vi "OceanOptics_30sec_img_while_scan.vi"() -> ()   [LabVIEW 2016]
uses:
  C:/Program Files/Ocean Optics/OmniDriver/OOI_HOME/NETOmniDriver-NET40.dll
  Program Files/Ocean Optics/OmniDriver/OOI_HOME/NETOmniDriver-NET40.dll
  <vilib>/DAQmx/create/channels.llb/DAQmx Create Channel (DO-Digital Output).vi
panel:
  in  "lastTriggerMilliseconds":i32
  in  "error in":errorcluster
  out "error out 2":errorcluster
  in  "Trigger":bool
  in  "Action B":bool
  out "getBufferCapacity":i32
  in  "read":bool
  in  "start":bool
  in  "abort":bool
  in  "stop":bool
  out "spectrum":cluster{"Y":dbl[], "Y":dbl[]}[](graph)
  out "getExternalTriggerMode":i32
  in  "clear":bool
  out "getNumberOfElements before readout":i32
  out "status":bool
  out "error out":errorcluster
  in  "integration time [us]":i32=100000
  # "Mode 3 = single trigger"
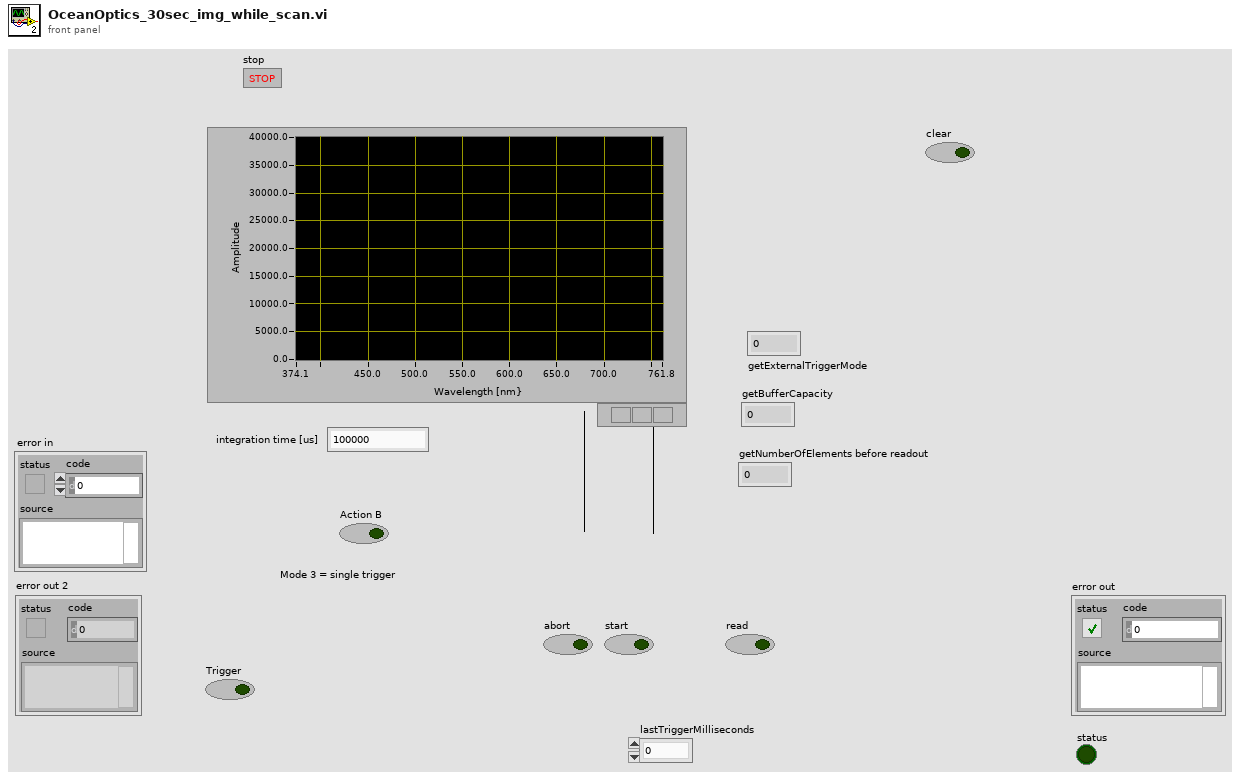
[diagram p1: front panel]
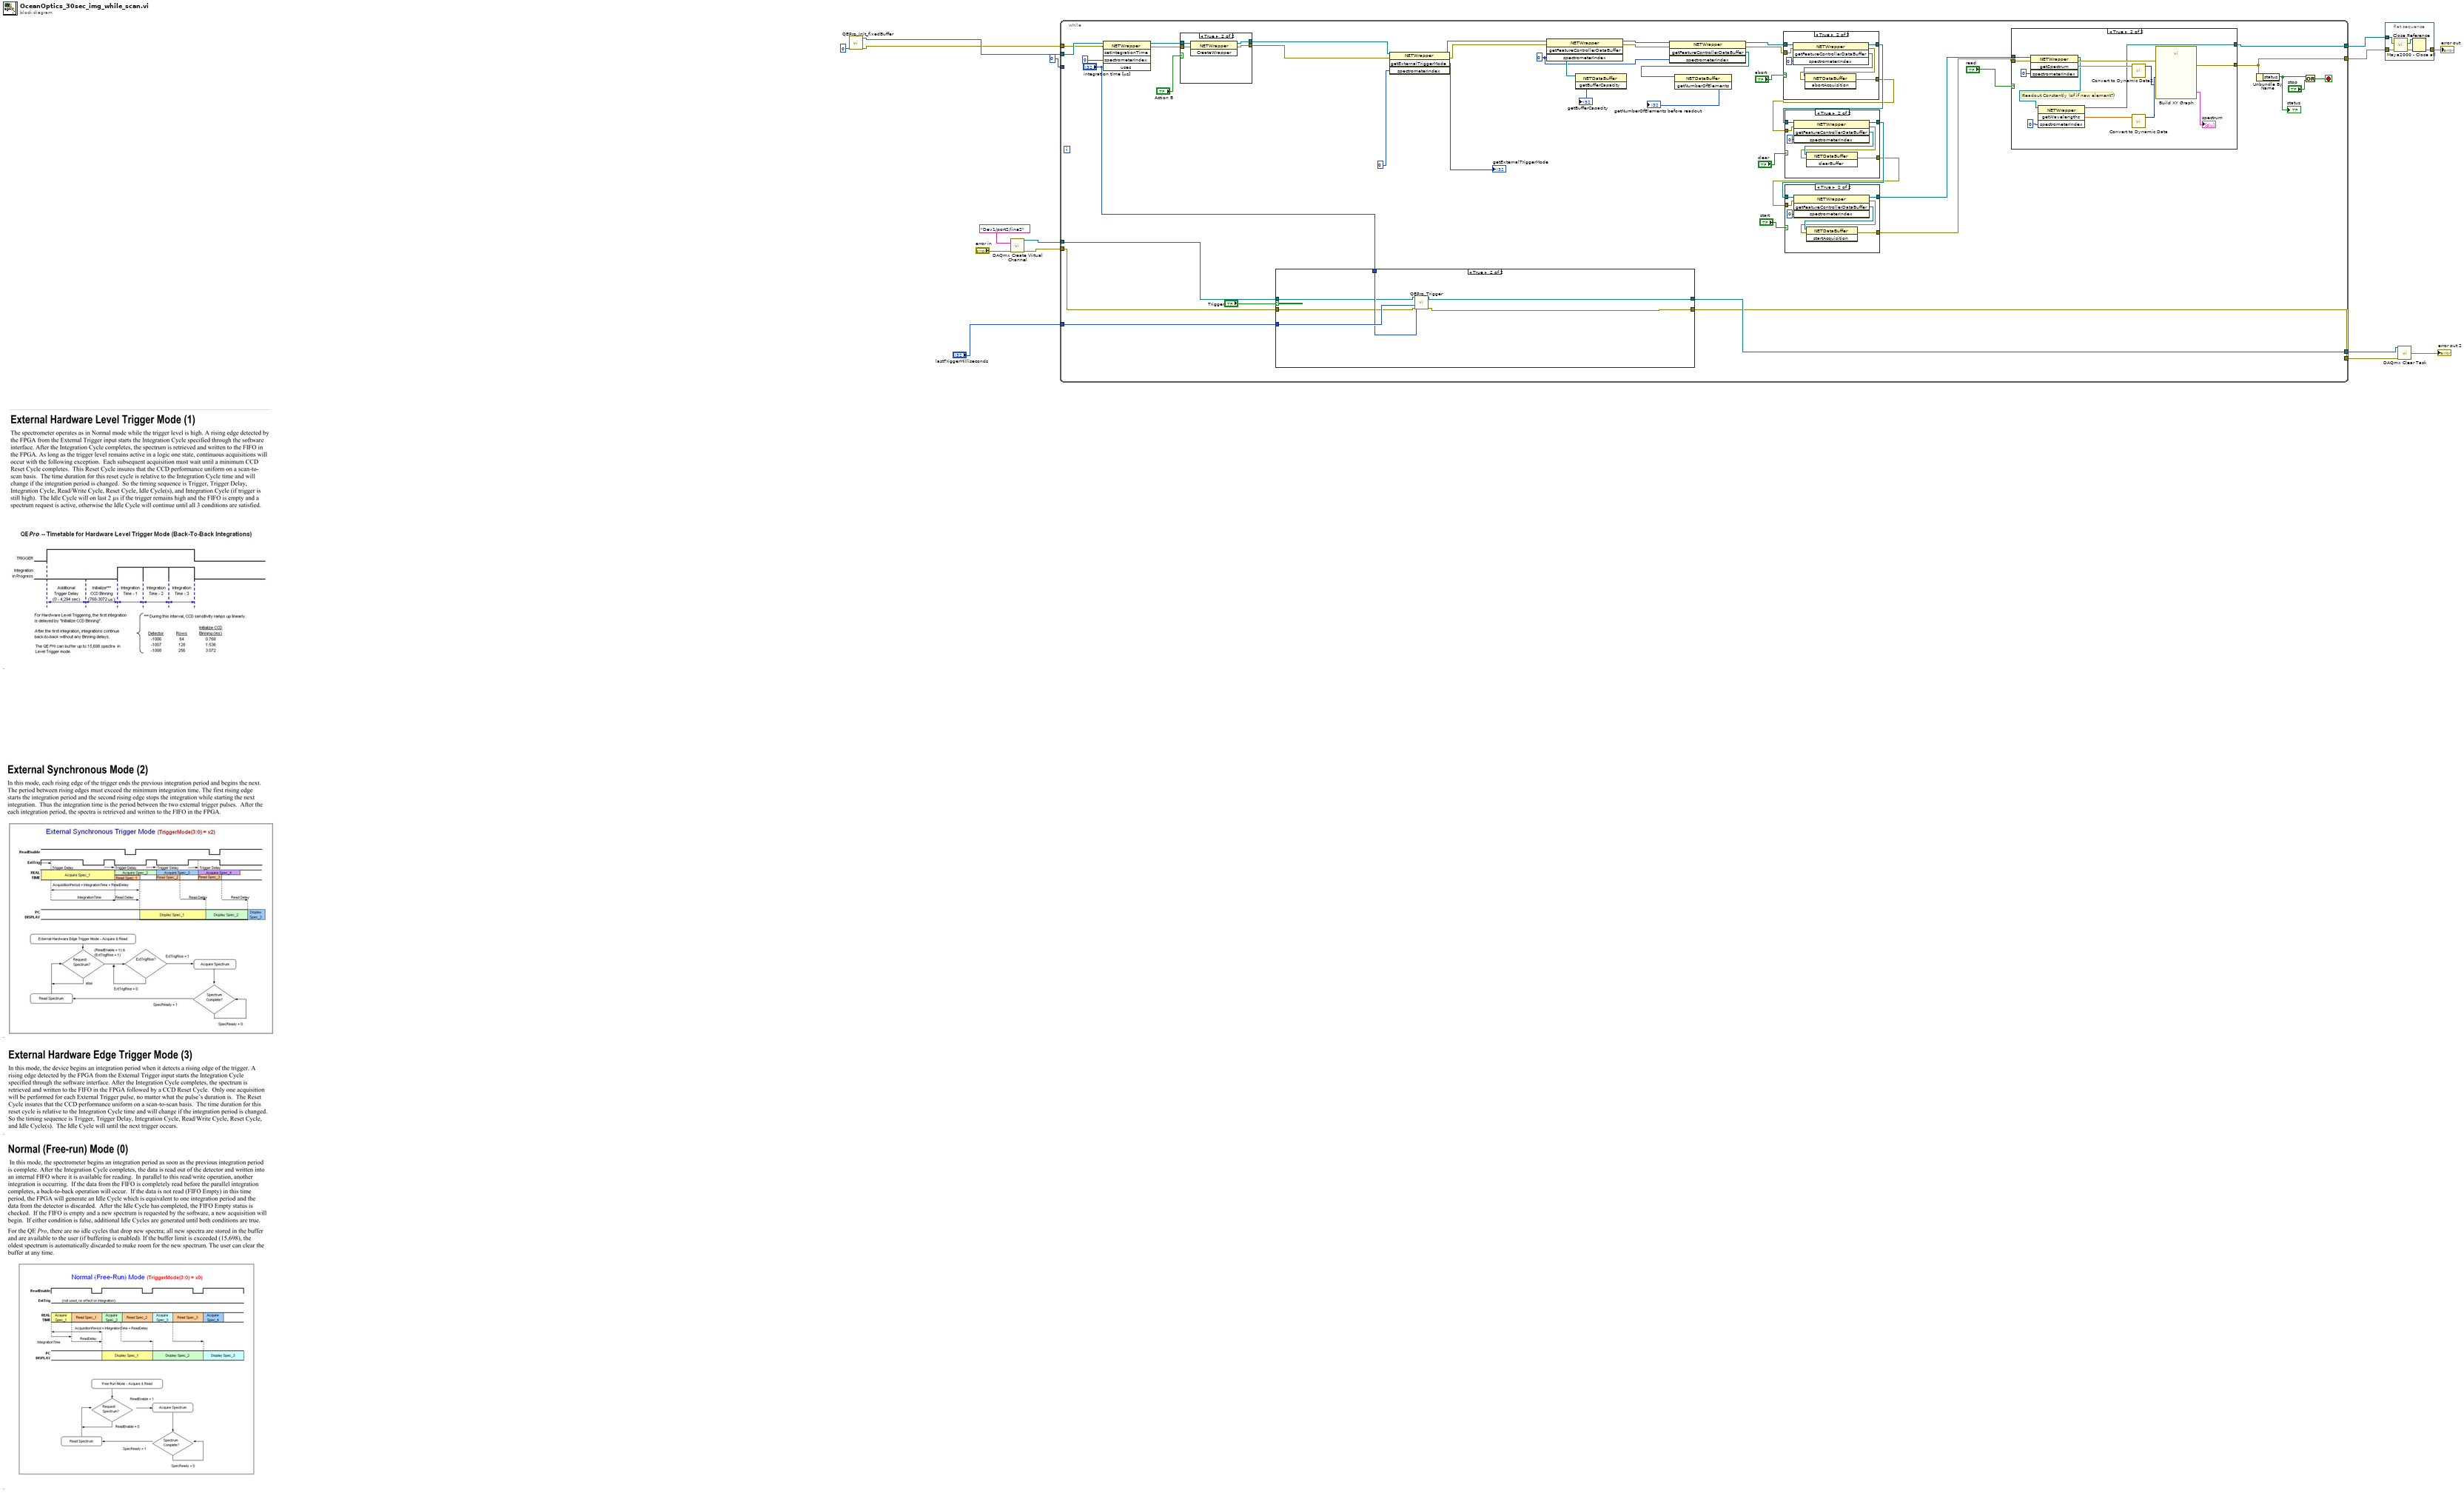
[diagram p0: block diagram]
diagram:
  n1 = call "QEPro_Init_fixedBuffer.vi"("Spectrometer Index"=0) -> ("error out"=w2:errorcluster, "reference out"=w5:refnum<k24>)  [unwired: 7 in, 2 out]
  n2 = call-poly <vilib>:"DAQmx Create Virtual Channel.vi"("lines"=tag "Dev1/port2/line2", "error in"="error in") -> ("task out"=w10:refnum<k21>, "error out"=w9:errorcluster)  [unwired: 12 in]
  n3 = while {
    tunnel: [w57] -> w15
    tunnel: 0 ("spectrometerIndex") -> [_]
    tunnel: w5 -> [w26]
    tunnel: w10 -> [w46]
    tunnel: w9 -> [w45]
    tunnel: [w44] -> w7
    tunnel: [w43] -> w6
    tunnel: [w25] -> w3
    tunnel: w2 -> [w24]
    tunnel: "lastTriggerMilliseconds" -> [w23]
    stop <- w56 stop-if-true
    w38 = 0 ("spectrometerIndex")
    n4 = invoke class="NETWrapper" method="setIntegrationTime"(reference=w26, error in=w24, "spectrometerIndex"=0 ("mode"), "usec"="integration time [us]") -> (reference out=w48:refnum<k24>, error out=w47:errorcluster)  [unwired: 1 in, 3 out]
    n5 = case shown="True" "Action B" {
      tunnel: w48 -> [w86 w90]
      tunnel: [w86 w89] -> w19
      tunnel: w47 -> [w85 w88]
      tunnel: [w85 w87] -> w18
      frame False {
      }
      frame True {
        n6 = invoke class="NETWrapper" method="CreateWrapper"(reference=w90, error in=w88) -> (reference out=w89:refnum<k24>, error out=w87:errorcluster)  [unwired: 1 in, 1 out]
      }
    }
    n7 = case shown="True" "Trigger" {
      tunnel: w46 -> [w78 w79]
      tunnel: w45 -> [w77 w80]
      tunnel: [w78 w84] -> w44
      tunnel: [w77 w83] -> w43
      tunnel: w23 -> [_ w82]
      tunnel: "integration time [us]" -> [_ w81]
      frame False {
      }
      frame True {
        n8 = call "QEPro_Trigger.vi"("task in"=w79, "integration time [us]"=w81, "lastTriggerMilliseconds"=w82, "error in"=w80) -> ("task out"=w84:refnum<k21>, "error out"=w83:errorcluster)  [unwired: 9 in, 1 out]
      }
    }
    n9 = invoke class="NETWrapper" method="getExternalTriggerMode"(reference=w19, error in=w18, "spectrometerIndex"=0) -> (reference out=w16:refnum<k24>, error out=w17:errorcluster, "getExternalTriggerMode"=→"getExternalTriggerMode":i32)  [unwired: 1 in, 1 out]
    n10 = invoke class="NETWrapper" method="getFeatureControllerDataBuffer"(reference=w16, error in=w17, "spectrometerIndex"=w38) -> (reference out=w40:refnum<k24>, error out=w39:errorcluster, "getFeatureControllerDataBuffer"=w54:refnum<k24>)  [unwired: 1 in, 1 out]
    n11 = invoke class="NETDataBuffer" method="getBufferCapacity"(reference=w54) -> ("getBufferCapacity"=→"getBufferCapacity":i32)  [unwired: 2 in, 2 out]
    n12 = invoke class="NETWrapper" method="getFeatureControllerDataBuffer"(reference=w40, error in=w39, "spectrometerIndex"=w38) -> (reference out=w37:refnum<k24>, error out=w36:errorcluster, "getFeatureControllerDataBuffer"=w41:refnum<k24>)  [unwired: 1 in, 1 out]
    n13 = invoke class="NETDataBuffer" method="getNumberOfElements"(reference=w41) -> ("getNumberOfElements"=→"getNumberOfElements before readout":i32)  [unwired: 2 in, 2 out]
    n14 = case shown="True" "abort" {
      tunnel: w37 -> [w106 w114]
      tunnel: [w106 w109] -> w31
      tunnel: [w107 w111] -> w28
      tunnel: w36 -> [w107 w110]
      frame False {
      }
      frame True {
        n15 = invoke class="NETWrapper" method="getFeatureControllerDataBuffer"(reference=w114, error in=w110, "spectrometerIndex"=0) -> (reference out=w109:refnum<k24>, error out=w112:errorcluster, "getFeatureControllerDataBuffer"=w113:refnum<k24>)  [unwired: 1 in, 1 out]
        n16 = invoke class="NETDataBuffer" method="abortAcquisition"(reference=w113, error in=w112) -> (error out=w111:errorcluster)  [unwired: 1 in, 2 out]
      }
    }
    n17 = case shown="True" "clear" {
      tunnel: w31 -> [w68 w76]
      tunnel: [w68 w71] -> w30
      tunnel: [w69 w73] -> w29
      tunnel: w28 -> [w69 w72]
      frame False {
      }
      frame True {
        n18 = invoke class="NETWrapper" method="getFeatureControllerDataBuffer"(reference=w76, error in=w72, "spectrometerIndex"=0) -> (reference out=w71:refnum<k24>, error out=w74:errorcluster, "getFeatureControllerDataBuffer"=w75:refnum<k24>)  [unwired: 1 in, 1 out]
        n19 = invoke class="NETDataBuffer" method="clearBuffer"(reference=w75, error in=w74) -> (error out=w73:errorcluster)  [unwired: 1 in, 2 out]
      }
    }
    n20 = case shown="True" "start" {
      tunnel: w30 -> [w59 w67]
      tunnel: [w59 w66] -> w32
      tunnel: [w60 w63] -> w27
      tunnel: w29 -> [w60 w62]
      frame False {
      }
      frame True {
        n21 = invoke class="NETWrapper" method="getFeatureControllerDataBuffer"(reference=w67, error in=w62, "spectrometerIndex"=0) -> (reference out=w66:refnum<k24>, error out=w64:errorcluster, "getFeatureControllerDataBuffer"=w65:refnum<k24>)  [unwired: 1 in, 1 out]
        n22 = invoke class="NETDataBuffer" method="startAcquisition"(reference=w65, error in=w64) -> (error out=w63:errorcluster)  [unwired: 1 in, 2 out]
      }
    }
    n23 = case shown="True" "read" {
      tunnel: [w91 w93] -> w25
      tunnel: [w92 w105] -> w57
      tunnel: w32 -> [w91 w97]
      tunnel: w27 -> [w92 w96]
      frame False {
      }
      frame True {
        # "Readout Constantly (of if new element?)"
        n24 = invoke class="NETWrapper" method="getSpectrum"(reference=w97, error in=w96, "spectrometerIndex"=0) -> (reference out=w94:refnum<k24>, error out=w95:errorcluster, "getSpectrum"=w99:dbl[])  [unwired: 1 in, 1 out]
        n25 = invoke class="NETWrapper" method="getWavelengths"(reference=w94, "spectrometerIndex"=0) -> (reference out=w93:refnum<k24>, "getWavelengths"=w103:dbl[])  [unwired: 2 in, 2 out]
        n26 = call "Convert to Dynamic Data2"("Array"=w99) -> ("Dynamic Data Type"=w100:dynamicdata)  [unwired: 3 in]
        n27 = call "Convert to Dynamic Data"("Array"=w103) -> ("Dynamic Data Type"=w101:dynamicdata)  [unwired: 3 in]
        n28 = call "Build XY Graph"("error in (no error)"=w95, "Y Input"=w100, "X Input"=w101) -> ("error out"=w105:errorcluster, "XY Graph"=→"spectrum":cluster{"X":dbl[], "Y":dbl[]}[])  [unwired: 7 in]
      }
    }
    n29 = Unbundle By Name(w57) -> ("status"=w51:bool)
    "status" <- w51
    n30 = Or(x=w51, y="stop") -> (x .or. y?=w56:bool)
  }
  n31 = flat-sequence {
    tunnel: w3 -> [w119]
    tunnel: w15 -> [w118]
    tunnel: [w117] -> w14
    frame #0 {
      n32 = call "Maya2000 - Close all.vi"("error in (no error)"=w118, "Maya reference in"=w119) -> ("error out"=w116:errorcluster, ".NET Refnum out"=w115:refnum<k24>)  [unwired: 8 in]
      n33 = Close Reference(reference=w115, error in (no error)=w116) -> (error out=w117:errorcluster)
    }
  }
  n34 = call <vilib>:"DAQmx Clear Task.vi"("task in"=w7, "error in"=w6) -> ("error out"=→"error out 2":errorcluster)  [unwired: 13 in]
  "error out" <- w14
